vi "StartData.vi"(8 "error in (no error)":errorcluster, 11 "Class In":refnum<class "SiemensDigitalEnergyMeter.lvclass">) -> (0 "error out":errorcluster, 3 "Class Out":refnum<class "SiemensDigitalEnergyMeter.lvclass">)   [LabVIEW 2018, in "SensorPlugins.lvlib" / "SiemensDigitalEnergyMeter.lvclass"]
doc: "This VI starts the retrieval of measurements from the Siemens Digital Energy Meter."
uses:
  SiemensDigitalEnergyMeter.lvclass
  SiemensDigitalEnergyMeter.lvclass/SiemensDigitalEnergyMeter.ctl
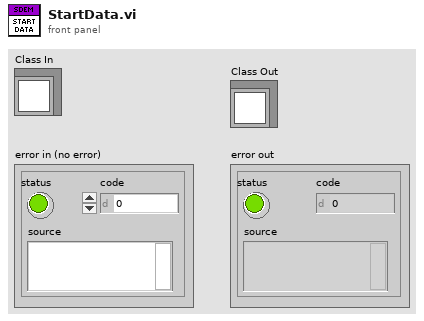
[diagram p1: front panel]
types:
  T1 = typedef "SensorPlugins.lvlib/SiemensDigitalEnergyMeter.lvclass/SiemensDigitalEnergyMeterControls.ctl" = cluster{"Measurement(s)":u16[], "Configuration Commands":string, "Use Measurement Commands Text Box?":bool, "Measurement Commands":string, "Connected?":bool, "Serial Number":string, "IP Address":string, "Port (502)":u16, "Unit ID":u8, "Serial Type":enum16{"RTU", "ASCII"}, "VISA Resource Name":refnum<visa-resource-name>, "Using TCP?":bool}[]
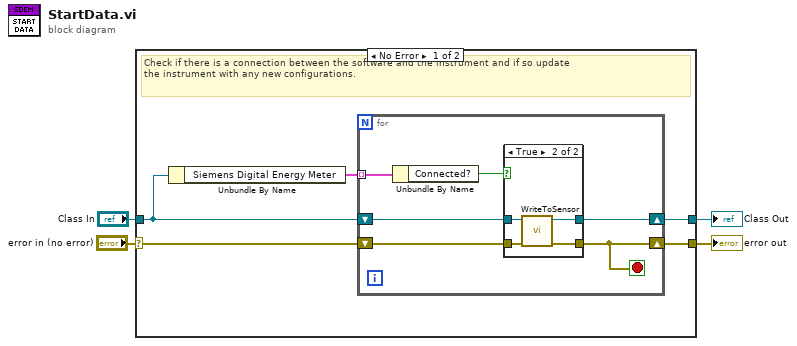
[diagram p0: block diagram]
diagram:
  n1 = case shown="No Error" "error in (no error)" {
    selector: "error in (no error)" -> [w9 w23]
    tunnel: [w8 w22] -> w3
    tunnel: [w7 w23] -> w2
    tunnel: "Class In" -> [w6 w22]
    frame No Error {
      # "Check if there is a connection between the software and the instrument and if so update\nthe instrument with any new configurations."
      n2 = Unbundle By Name(w6) -> ("Siemens Digital Energy Meter"=w5:T1)
      n3 = for {
        shift-right: [w10] -> w7
        shift-left: w9 -> [w15]
        shift-right: [w14] -> w8
        shift-left: w6 -> [w13]
        tunnel: w5 -> [w12] mode=indexing
        stop <- w10 stop-if-true
        n4 = Unbundle By Name(w12) -> ("Connected?"=w11:bool)
        n5 = case shown="True" w11 {
          tunnel: w15 -> [w16 w21]
          tunnel: [w17 w20] -> w14
          tunnel: [w16 w19] -> w10
          tunnel: w13 -> [w17 w18]
          frame False {
          }
          frame True {
            n6 = call-dynamic "WriteToSensor.vi"("error in (no error)"=w21, "SiemensDigitalEnergyMeter in"=w18) -> ("error out"=w19:errorcluster, "SiemensDigitalEnergyMeter out"=w20:refnum<class "SiemensDigitalEnergyMeter.lvclass">)  [unwired: 8 in]
          }
        }
      }
    }
    frame Error {
    }
  }
  "Class Out" <- w3
  "error out" <- w2
